vi "HTTP_Accel_Reader.vi"() -> ()   [LabVIEW 2021]
uses:
  <vilib>/myRIO/Instrument Drivers/Onboard Devices/Accelerometer/typedefs/Accelerometer Reference.ctl
  <vilib>/myRIO/Common/Instrument Driver Framework/Utilities/typedefs/myRIO Generic Hardware Reference.ctl
  <vilib>/myRIO/Common/Instrument Driver Framework/Utilities/typedefs/Hardware Version Enum.ctl
  <vilib>/myRIO/Common/Instrument Driver Framework/Utilities/typedefs/myRIO v1.0 Reference.ctl
  <vilib>/myRIO/Common/Instrument Driver Framework/Utilities/typedefs/Generic FPGA Reference.ctl
  <vilib>/myRIO/Common/Instrument Driver Framework/myRIO v1.0/Accelerometer/typedefs/Accelerometer Channels List.ctl
  <vilib>/myRIO/Common/Instrument Driver Framework/myRIO v1.0/Accelerometer/typedefs/Accelerometer Channels Enum.ctl
  <vilib>/userDefined/High Color/nirio_resource_hc.ctl
  <vilib>/myRIO/Instrument Drivers/Onboard IO/AI/typedefs/AI Reference.ctl
  <vilib>/myRIO/Common/Instrument Driver Framework/myRIO v1.0/AI/typedefs/AI Channels List.ctl
  <vilib>/myRIO/Common/Instrument Driver Framework/myRIO v1.0/AI/typedefs/AI Channels Enum.ctl
  <vilib>/myRIO/Common/Instrument Driver Framework/Utilities/typedefs/Analog Scaling Constants List.ctl
  <vilib>/myRIO/Common/Instrument Driver Framework/Utilities/typedefs/Analog Scaling Constants.ctl
  <vilib>/myRIO/Instrument Drivers/Onboard IO/DIO/typedefs/DIO Reference.ctl
  <vilib>/myRIO/Common/Instrument Driver Framework/myRIO v1.0/DIO/typedefs/DIO Channels List.ctl
  <vilib>/myRIO/Common/Instrument Driver Framework/myRIO v1.0/DIO/typedefs/DIO Channels Enum.ctl
  <vilib>/myRIO/Common/Instrument Driver Framework/Utilities/vis/Is FPGA Ref Available.vi
  <vilib>/myRIO/Common/Instrument Driver Framework/myRIO v1.0/AI/vis/myRIO v1.1 Open AI.vi
  <vilib>/myRIO/Instrument Drivers/Onboard IO/AI/vis/Read.vi
  <vilib>/myRIO/Common/Instrument Driver Framework/myRIO v1.0/Accelerometer/vis/myRIO v1.1 Open Accelerometer.vi
  <vilib>/myRIO/Instrument Drivers/Onboard Devices/Accelerometer/vis/Read.vi
  <vilib>/myRIO/Common/Instrument Driver Framework/myRIO v1.0/DIO/vis/myRIO v1.1 Open DIO.vi
  <vilib>/myRIO/Instrument Drivers/Onboard IO/DIO/vis/Write.vi
  <vilib>/myRIO/Common/Instrument Driver Framework/Utilities/vis/Validate Channels.vi
  <vilib>/myRIO/Common/Instrument Driver Framework/myRIO v1.0/AI/vis/myRIO v1.0 Reserve AI.vi
  <vilib>/myRIO/Common/Instrument Driver Framework/myRIO v1.0/Accelerometer/vis/myRIO v1.0 Reserve Accelerometer.vi
  <vilib>/myRIO/Common/Instrument Driver Framework/myRIO v1.0/DIO/vis/myRIO v1.0 Reserve DIO.vi
  <vilib>/myRIO/Common/Instrument Driver Framework/myRIO v1.0/AI/vis/myRIO v1.0 Build MUX Configuration AI.vi
  <vilib>/myRIO/Common/Instrument Driver Framework/myRIO v1.0/Resource Manager/vis/myRIO v1.0 Reserve Channel List.vi
  <vilib>/myRIO/Common/Instrument Driver Framework/myRIO v1.0/Accelerometer/vis/myRIO v1.0 Build MUX Configuration Accelerometer.vi
  <vilib>/myRIO/Common/Instrument Driver Framework/myRIO v1.0/DIO/vis/myRIO v1.0 Build MUX Configuration DIO.vi
  <vilib>/myRIO/Common/Instrument Driver Framework/myRIO v1.0/Resource Manager/vis/myRIO v1.0 Reserve Channel.vi
  <vilib>/myRIO/Common/Instrument Driver Framework/myRIO v1.0/Resource Manager/vis/myRIO v1.0 Unreserve Channel.vi
  <vilib>/myRIO/Common/Instrument Driver Framework/myRIO v1.0/Resource Manager/vis/myRIO v1.0 Create Configuration List.vi
  <vilib>/myRIO/Common/Instrument Driver Framework/myRIO v1.0/Resource Manager/vis/myRIO v1.0 Build Mutex Name.vi
  <vilib>/Utility/VariantDataType/GetNumericInfo.vi
  <vilib>/Utility/error.llb/Error Cluster From Error Code.vi
  <vilib>/myRIO/Common/Instrument Driver Framework/myRIO v1.0/myRIO v1.1 Open.vi
  <vilib>/myRIO/Common/Instrument Driver Framework/myRIO v1.0/Accelerometer/vis/myRIO v1.0 Get Scaling Constant Accelerometer.vi
  <vilib>/myRIO/Common/Instrument Driver Framework/Utilities/vis/IO Manager.vi
  <vilib>/myRIO/Common/Instrument Driver Framework/Utilities/vis/Configuration Manager.vi
  <vilib>/myRIO/Common/Instrument Driver Framework/myRIO v1.0/myRIO v1.0 Close.vi
  <vilib>/myRIO/Common/Instrument Driver Framework/myRIO v1.0/Accelerometer/vis/myRIO v1.0 Read Accelerometer.vi
  <vilib>/myRIO/Common/Instrument Driver Framework/myRIO v1.0/AI/vis/myRIO v1.0 Get Scaling Constants AI.vi
  <vilib>/myRIO/Common/Instrument Driver Framework/myRIO v1.0/AI/vis/myRIO v1.0 Read AI.vi
  <vilib>/myRIO/Common/Instrument Driver Framework/myRIO v1.0/Resource Manager/vis/myRIO v1.0 Configure IO.vi
  <vilib>/myRIO/Common/Instrument Driver Framework/myRIO v1.0/DIO/vis/myRIO v1.0 Write DIO.vi
  <vilib>/httpClient/POSTBuffer.vi
  <vilib>/myRIO/Express VI/Onboard Devices/Accelerometer/Accelerometer Express VI.xnode
  <vilib>/myRIO/Instrument Drivers/Onboard Devices/Accelerometer/vis/myRIO Accelerometer Open.xnode
  <vilib>/myRIO/Express VI/Onboard IO/AI/AI Express VI.xnode
  <vilib>/myRIO/Instrument Drivers/Onboard IO/AI/vis/myRIO AI Open.xnode
  <vilib>/myRIO/Express VI/Onboard IO/DO/DO Express VI.xnode
  <vilib>/myRIO/Instrument Drivers/Onboard IO/DIO/vis/myRIO DIO Open.xnode
  <vilib>/myRIO/Instrument Drivers/Onboard Devices/Accelerometer/Accelerometer.lvlib
  <vilib>/myRIO/Instrument Drivers/Onboard IO/DIO/DIO.lvlib
  <vilib>/httpClient/LabVIEWHTTPClient.lvlib
  <vilib>/myRIO/Instrument Drivers/Onboard IO/AI/AI.lvlib
panel:
  out "element":string
  out "Address2":string
  out "Address1":string
  in  "stop 2":bool
  out "txt":string
  out "txt 2":string
  out "error out 3":errorcluster
  out "error out 2":errorcluster
  out "A/AI3 (Pin 9)":dbl
  out "A/AI0 (Pin 3)":dbl
  out "output variable":dbl
  out "date string":string
  out "error out":errorcluster
  in  "stop":bool
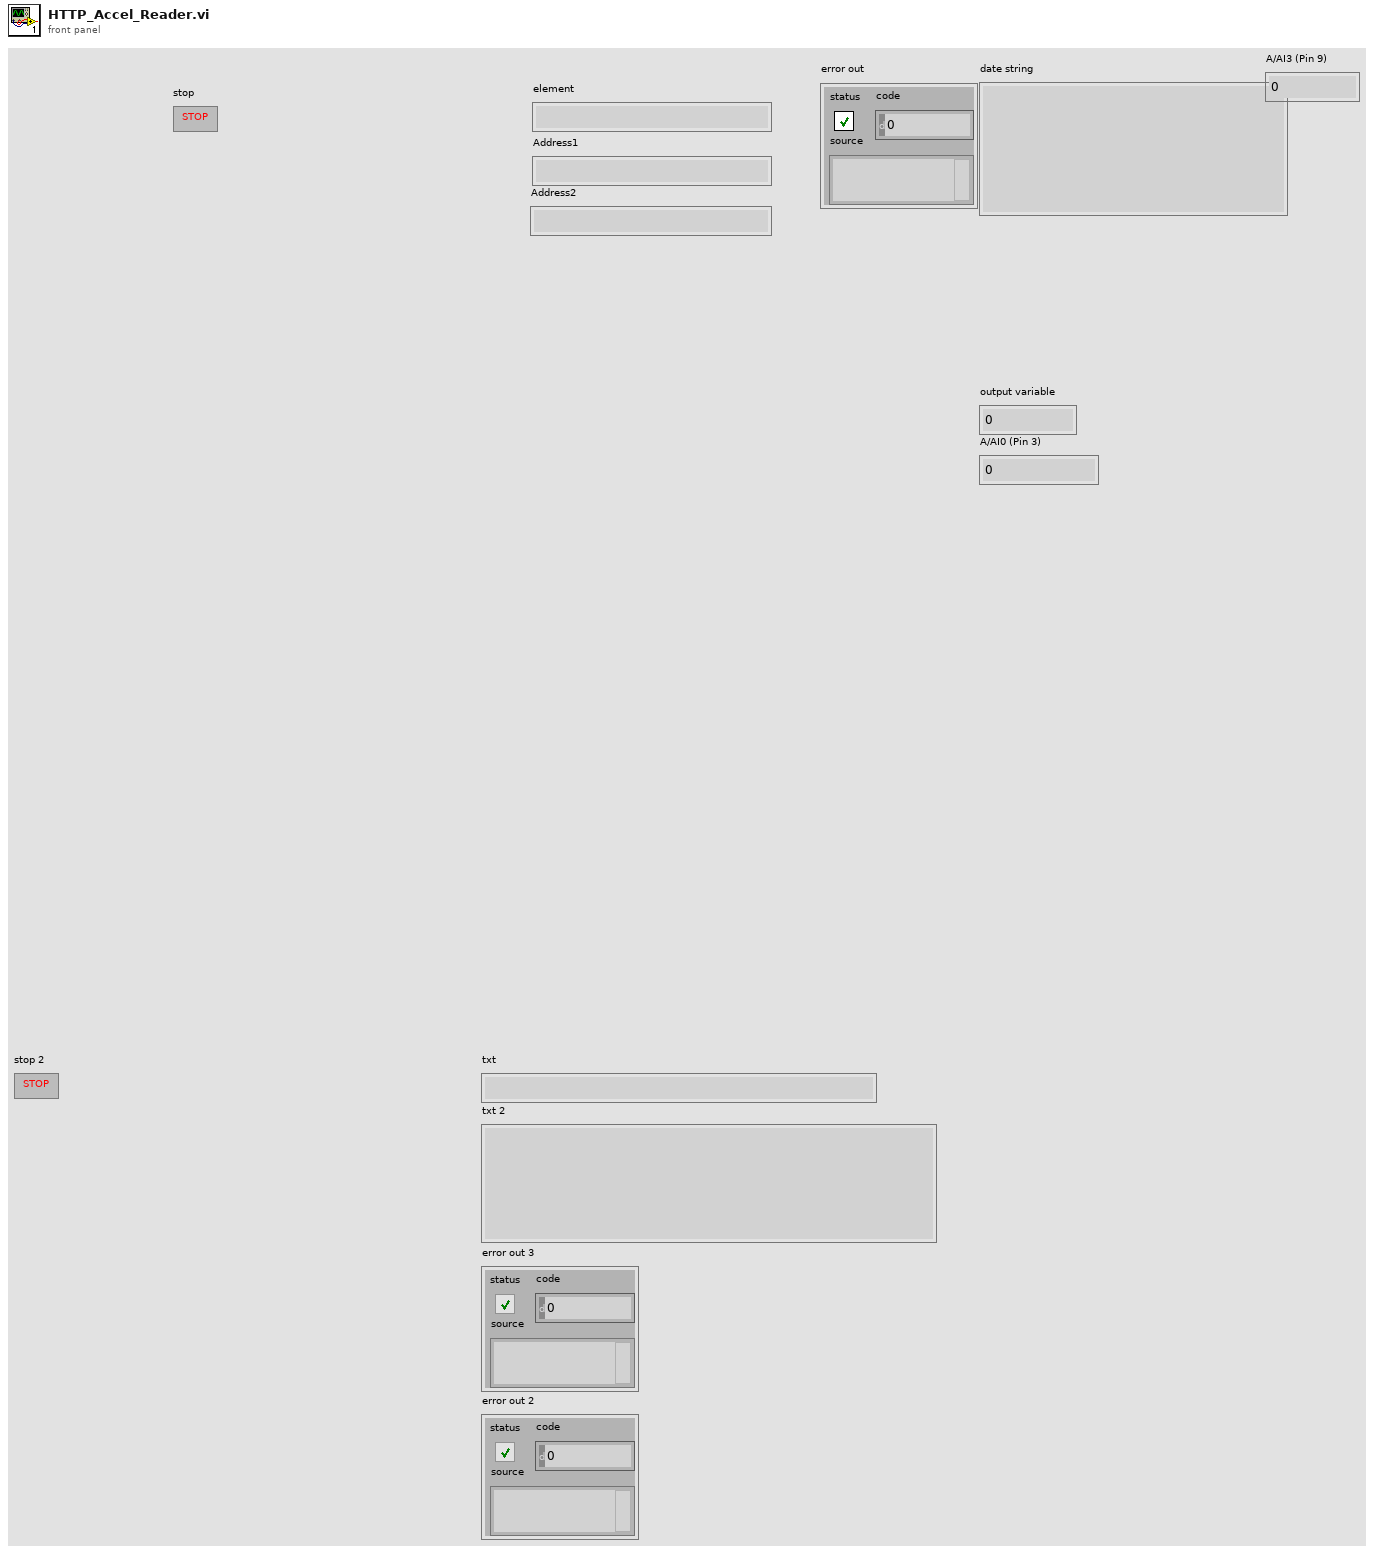
[diagram p1: front panel]
types:
  T1 = typedef "LabVIEWHTTPClient.lvlib/ClientHandle.ctl" = refnum<k1>
  T2 = typedef "DIO.lvlib/DIO Reference.ctl" = cluster{"myRIO Reference":T3, "DIO Channels List":T7}
  T3 = typedef "myRIO Generic Hardware Reference.ctl" = cluster{"myRIO Model":T4, "myRIO Hardware Reference":T5}
  T4 = typedef "Hardware Version Enum.ctl" = enum16{"Unknown", "myRIO-1900", "myRIO-1950", "roboRIO", "NI ELVIS RIO CM", "ELVIS III"}
  T5 = typedef "myRIO v1.0 Reference.ctl" = cluster{"Generic FPGA Reference":T6, "Allow multiple opens":bool}
  T6 = typedef "Generic FPGA Reference.ctl" = refnum<k20>
  T7 = typedef "DIO Channels List.ctl" = T8[]
  T8 = typedef "DIO Channels Enum.ctl" = enum16{"Not Connected", "C/DIO0", "C/DIO1", "C/DIO2", "C/DIO3", "C/DIO4", "C/DIO5", "C/DIO6", "C/DIO7", "A/DIO0", "A/DIO1", "A/DIO2", "A/DIO3", "A/DIO4", "A/DIO5", "A/DIO6", "A/DIO7", "A/DIO8", "A/DIO9", "A/DIO10", "A/DIO11", "A/DIO12", "A/DIO13", "A/DIO14", "A/DIO15", "A/DIO16", "A/DIO17", "A/DIO18", "A/DIO19", "B/DIO0", "B/DIO1", "B/DIO2", "B/DIO3", "B/DIO4", "B/DIO5", "B/DIO6", "B/DIO7", "B/DIO8", "B/DIO9", "B/DIO10", "B/DIO11", "B/DIO12", "B/DIO13", "B/DIO14", "B/DIO15", "B/DIO16", "B/DIO17", "B/DIO18", "B/DIO19", "LED0", "LED1", "LED2", "LED3", "Button0", "DIO/DIO0", "DIO/DIO1", "DIO/DIO2", "DIO/DIO3", "DIO/DIO4", "DIO/DIO5", "DIO/DIO6", "DIO/DIO7", "DIO/DIO8", "DIO/DIO9", "SPI/CS0", "SPI/CS1", "SPI/CS2", "SPI/CS3", "LED RADIO (Green)", "LED RADIO (Red)", "LED COMM (Green)", "LED COMM (Red)", "LED MODE (Green)", "LED MODE (Red)"}
  T9 = typedef "nirio_resource_hc.ctl" = tag
  T10 = typedef "AI.lvlib/AI Reference.ctl" = cluster{"myRIO Reference":T3, "AI Channels List":T11, "AI Scaling Constants List":T13}
  T11 = typedef "AI Channels List.ctl" = T12[]
  T12 = typedef "AI Channels Enum.ctl" = enum16{"Not Connected", "AudioIn/Left", "AudioIn/Right", "C/AI0", "C/AI1", "A/AI0", "A/AI1", "A/AI2", "A/AI3", "A/AI4", "A/AI5", "A/AI6", "A/AI7", "B/AI0", "B/AI1", "B/AI2", "B/AI3", "B/AI4", "B/AI5", "B/AI6", "B/AI7", "AI/AI0", "AI/AI1", "AI/AI2", "AI/AI3", "A/AI0 (DIFF)", "A/AI1 (DIFF)", "A/AI2 (DIFF)", "A/AI3 (DIFF)", "B/AI0 (DIFF)", "B/AI1 (DIFF)", "B/AI2 (DIFF)", "B/AI3 (DIFF)"}
  T13 = typedef "Analog Scaling Constants List.ctl" = T14[]
  T14 = typedef "Analog Scaling Constants.ctl" = cluster{"LSB Weight (Volts)":dbl, "Offset (Volts)":dbl, "Signed?":bool}
  T15 = typedef "Accelerometer.lvlib/Accelerometer Reference.ctl" = cluster{"myRIO Reference":T3, "Accelerometer Channels List":T16, "LSB Weight":dbl}
  T16 = typedef "Accelerometer Channels List.ctl" = T17[]
  T17 = typedef "Accelerometer Channels Enum.ctl" = enum16{"Not Connected", "X-Axis", "Y-Axis", "Z-Axis"}
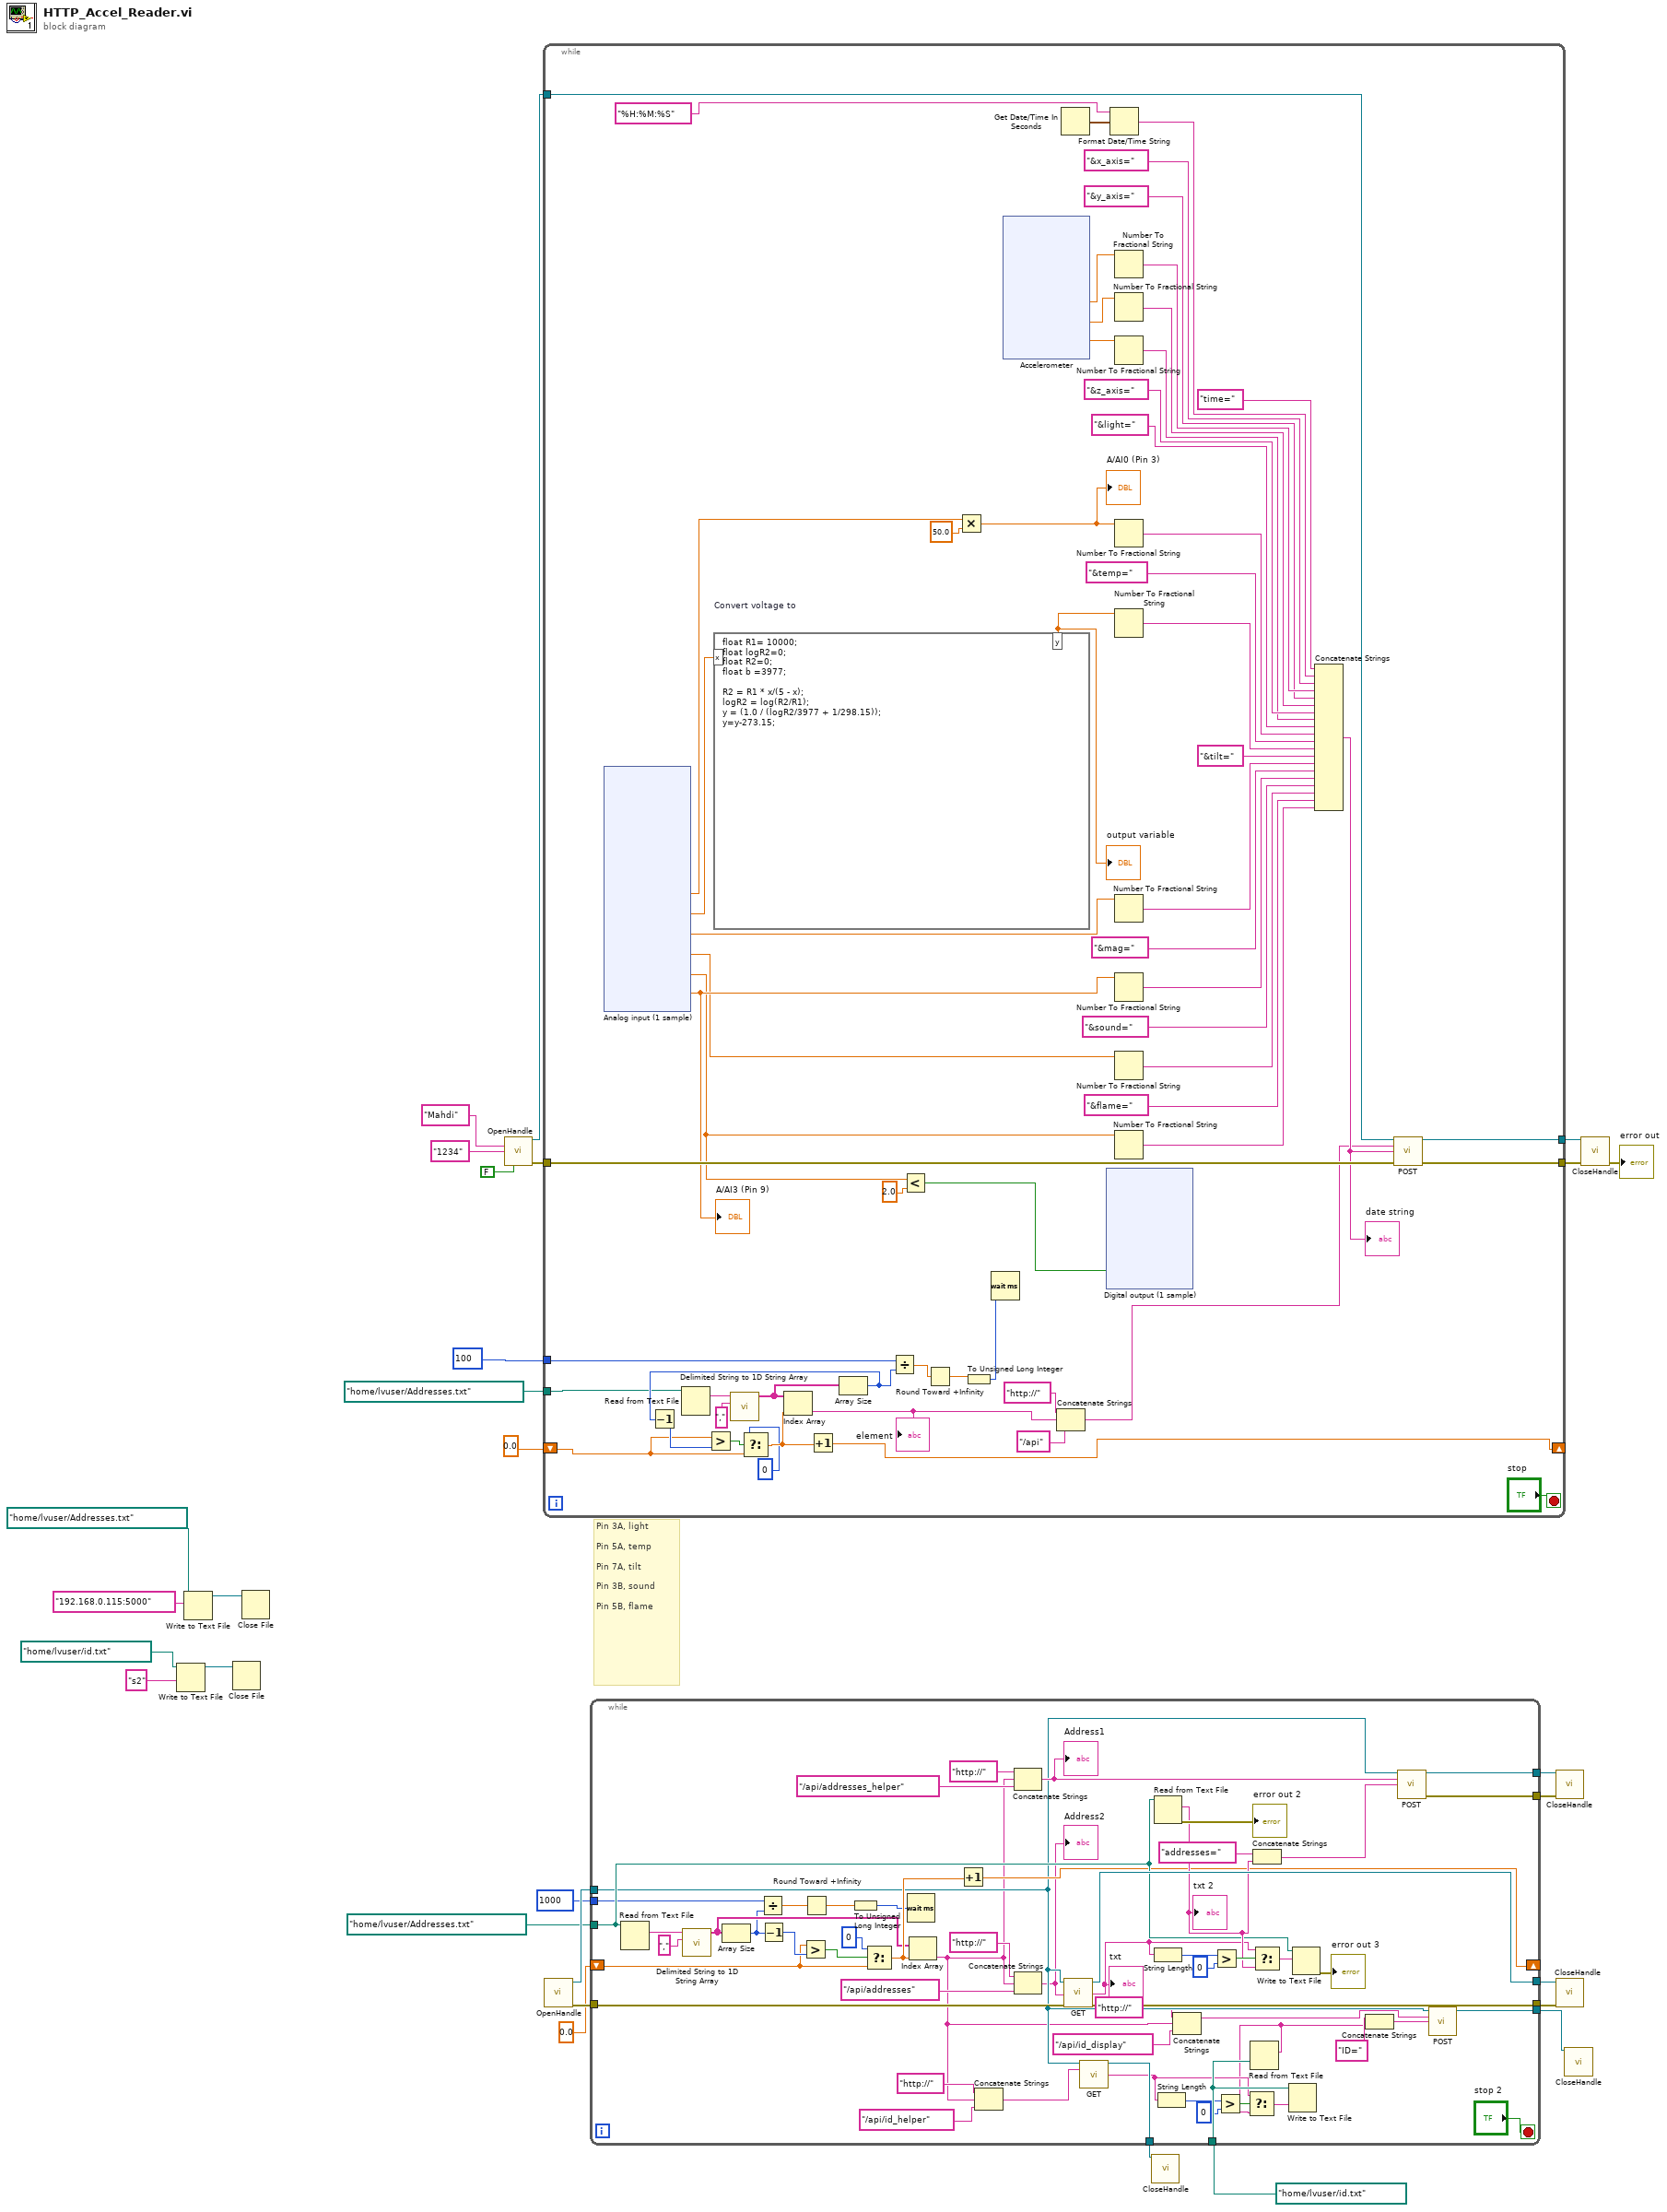
[diagram p0: block diagram]
diagram:
  # "Pin 3A, light\n\nPin 5A, temp\n\nPin 7A, tilt\n\nPin 3B, sound\n\nPin 5B, flame"
  n1 = Write to Text File(file (use dialog)=path "/home/lvuser/id.txt" ("file path (use dialog)"), text="s2") -> (refnum out=w3:refnum<file>)  [unwired: 2 in, 2 out]
  n2 = Write to Text File(file (use dialog)=path "/home/lvuser/Addresses.txt" ("file path (use dialog)"), text="192.168.0.115:5000") -> (refnum out=w4:refnum<file>)  [unwired: 2 in, 2 out]
  n3 = Close File(refnum=w3) -> ()  [unwired: 1 in, 2 out]
  n4 = Close File(refnum=w4) -> ()  [unwired: 1 in, 2 out]
  n5 = call <vilib>:"OpenHandle.vi"("username"="Mahdi", "password"="1234", "verify server(true)"=FALSE) -> ("client handle out"=w27:T1, "error out"=w26:errorcluster)  [unwired: 11 in]
  n6 = while {
    tunnel: w27 -> [w81]
    tunnel: w26 -> [w78]
    tunnel: [w79] -> w23
    tunnel: [w80] -> w24
    tunnel: u32 100 ("millisecond timer value") -> [w34]
    tunnel: path "/home/lvuser/Addresses.txt" ("file path (use dialog)") -> [w33]
    shift-right: [w31] -> _
    shift-left: 0.0 -> [w32]
    stop <- "stop" stop-if-true
    n7 = xnode "Analog input (1 sample)"() -> ("A/AI0 (Pin 3)"=w63:dbl, "A/AI1 (Pin 5)"=w64:dbl, "A/AI2 (Pin 7)"=w60:dbl, "B/AI0 (Pin 3)"=w55:dbl, "B/AI1 (Pin 5)"=w51:dbl, "A/AI3 (Pin 9)"=w57:dbl)  [unwired: 1 in, 1 out]
    "A/AI3 (Pin 9)" <- w57
    n8 = Read from Text File(file (use dialog)=w33) -> (text=w41:string)  [unwired: 3 in, 3 out]
    n9 = formula code="float R1= 10000; \nfloat logR2=0; \nfloat R2=0;\nfloat b =3977;\n\nR2 = R1 * x/(5 - x); \nlogR2 = log(R2/R1);\ny = (1.0 / (logR2/3977 + 1/298.15)); \ny=y-273.15;" "Convert voltage to"("x"=w64) -> ("y"=w69:dbl)
    "output variable" <- w69
    n10 = call <vilib>:"Delimited String to 1D String Array.vi"("delimiter"=",", "delimited string"=w41) -> ("string array"=w43:string[])  [unwired: 9 in]
    n11 = Array Size(array=w43) -> (size(s)=w35:i32)
    n12 = Decrement(x=w35) -> (x-1=w47:i32)
    n13 = Greater?(x=w32, y=w47) -> (0:w46:bool)
    n14 = Select(t=u32 0, s=w46, f=w32) -> (s? t:f=w48:dbl)
    n15 = Index Array(array=w43, index=w48) -> (element=w42:string)
    "element" <- w42
    n16 = Increment(x=w48) -> (x+1=w31:dbl)
    n17 = Divide(x=w34, y=w35) -> (x/y=w45:dbl)
    n18 = Less?(x=w51, y=2.0) -> (x < y?=w49:bool)
    n19 = Round Toward +Infinity(x=w45) -> (ceil(x): smallest int >= x=w44:dbl)
    n20 = Multiply(x=w63, y=50.0) -> (x*y=w70:dbl)
    "A/AI0 (Pin 3)" <- w70
    n21 = To Unsigned Long Integer(number=w44) -> (unsigned 32bit integer=w36:u32)
    n22 = Wait (ms)(milliseconds to wait=w36) -> ()  [unwired: 1 out]
    n23 = xnode "Accelerometer"() -> ("X-Axis"=w85:dbl, "Y-Axis"=w86:dbl, "Z-Axis"=w87:dbl)  [unwired: 1 in, 1 out]
    n24 = Concatenate Strings("http://" ("string"), w42, "/api" ("string")) -> (w30:string)
    n25 = Get Date/Time In Seconds() -> (seconds since 1Jan1904=w75:timestamp)
    n26 = xnode "Digital output (1 sample)"("B/DIO0 (Pin 11)"=w49) -> ()  [unwired: 1 in, 1 out]
    n27 = Format Date/Time String(time format string (%c)="%H:%M:%S", seconds (now)=w75) -> (date/time string=w74:string)  [unwired: 1 in]
    n28 = Number To Fractional String(number=w85) -> (F-format string=w88:string)  [unwired: 3 in]
    n29 = Number To Fractional String(number=w86) -> (F-format string=w89:string)  [unwired: 3 in]
    n30 = Number To Fractional String(number=w87) -> (F-format string=w72:string)  [unwired: 3 in]
    n31 = Number To Fractional String(number=w70) -> (F-format string=w67:string)  [unwired: 3 in]
    n32 = Number To Fractional String(number=w69) -> (F-format string=w66:string)  [unwired: 3 in]
    n33 = Number To Fractional String(number=w60) -> (F-format string=w61:string)  [unwired: 3 in]
    n34 = Number To Fractional String(number=w57) -> (F-format string=w58:string)  [unwired: 3 in]
    n35 = Number To Fractional String(number=w55) -> (F-format string=w54:string)  [unwired: 3 in]
    n36 = Number To Fractional String(number=w51) -> (F-format string=w53:string)  [unwired: 3 in]
    n37 = Concatenate Strings("time=" ("string"), w74, "&x_axis=", w88, "&y_axis=", w89, "&z_axis=", w72, "&light=", w67, "&temp=", w66, "&tilt=", w61, "&mag=", w58, "&sound=", w54, "&flame=", w53) -> (w76:string)
    "date string" <- w76
    n38 = call-poly <vilib>:"POST.vi"("client handle"=w81, "url"=w30, "buffer"=w76, "error in (no error)"=w78) -> ("client handle out"=w80:T1, "error out"=w79:errorcluster)  [unwired: 8 in, 2 out]
  }
  n39 = call <vilib>:"OpenHandle.vi"() -> ("client handle out"=w21:T1, "error out"=w20:errorcluster)  [unwired: 14 in]
  n40 = while {
    tunnel: path "/home/lvuser/Addresses.txt" ("file path (use dialog)") -> [w235]
    tunnel: w21 -> [w221]
    tunnel: w20 -> [w261]
    tunnel: [w260] -> w19
    tunnel: [w259] -> w18
    tunnel: [w258] -> w17
    tunnel: [w257] -> w16
    tunnel: u32 1000 ("millisecond timer value") -> [w234]
    shift-right: [w230] -> _
    shift-left: 0.0 -> [w231]
    tunnel: path "/home/lvuser/id.txt" ("file path (use dialog)") -> [w228]
    tunnel: [w222] -> w8
    tunnel: [w220] -> w7
    stop <- "stop 2" stop-if-true
    n41 = Read from Text File(file (use dialog)=w235) -> (text=w242:string)  [unwired: 3 in, 3 out]
    n42 = call <vilib>:"Delimited String to 1D String Array.vi"("delimiter"=",", "delimited string"=w242) -> ("string array"=w243:string[])  [unwired: 9 in]
    n43 = Array Size(array=w243) -> (size(s)=w229:i32)
    n44 = Divide(x=w234, y=w229) -> (x/y=w245:dbl)
    n45 = Decrement(x=w229) -> (x-1=w247:i32)
    n46 = Greater?(x=w231, y=w247) -> (0:w246:bool)
    n47 = Round Toward +Infinity(x=w245) -> (ceil(x): smallest int >= x=w244:dbl)
    n48 = To Unsigned Long Integer(number=w244) -> (unsigned 32bit integer=w233:u32)
    n49 = Select(t=u32 0, s=w246, f=w231) -> (s? t:f=w248:dbl)
    n50 = Wait (ms)(milliseconds to wait=w233) -> ()  [unwired: 1 out]
    n51 = Index Array(array=w243, index=w248) -> (element=w209:string)
    n52 = Increment(x=w248) -> (x+1=w230:dbl)
    n53 = Concatenate Strings("http://" ("string"), w209, "/api/id_helper" ("string")) -> (w213:string)
    n54 = Concatenate Strings("http://" ("string"), w209, "/api/addresses_helper" ("string")) -> (w232:string)
    "Address1" <- w232
    n55 = Concatenate Strings("http://" ("string"), w209, "/api/addresses" ("string")) -> (w214:string)
    "Address2" <- w214
    n56 = call <vilib>:"GET.vi"("client handle"=w221, "url"=w214, "error in (no error)"=w261) -> ("client handle out"=w259:T1, "body"=w226:string, "error out"=w260:errorcluster)  [unwired: 9 in, 1 out]
    "txt" <- w226
    n57 = call <vilib>:"GET.vi"("client handle"=w221, "url"=w213) -> ("client handle out"=w220:T1, "body"=w215:string)  [unwired: 10 in, 2 out]
    n58 = Read from Text File(file (use dialog)=w235) -> (text=w249:string, error out=→"error out 2":errorcluster)  [unwired: 3 in, 2 out]
    "txt 2" <- w249
    n59 = String Length(string=w226) -> (length=w252:i32)
    n60 = String Length(string=w215) -> (length=w219:i32)
    n61 = Concatenate Strings("http://" ("string"), w209, "/api/id_display" ("string")) -> (w210:string)
    n62 = Greater?(x=w252, y=0) -> (0:w251:bool)
    n63 = Greater?(x=w219, y=0) -> (0:w218:bool)
    n64 = Read from Text File(file (use dialog)=w228) -> (text=w207:string)  [unwired: 3 in, 3 out]
    n65 = Select(t=w215, s=w218, f=w207) -> (s? t:f=w216:string)
    n66 = Concatenate Strings("addresses=" ("string"), w249) -> (w255:string)
    n67 = Select(t=w226, s=w251, f=w249) -> (s? t:f=w227:string)
    n68 = Write to Text File(file (use dialog)=w228, text=w216) -> ()  [unwired: 2 in, 3 out]
    n69 = Write to Text File(file (use dialog)=w235, text=w227) -> (error out=→"error out 3":errorcluster)  [unwired: 2 in, 2 out]
    n70 = Concatenate Strings("ID=" ("string"), w207) -> (w223:string)
    n71 = call-poly <vilib>:"POST.vi"("client handle"=w221, "url"=w232, "buffer"=w255) -> ("client handle out"=w257:T1, "error out"=w258:errorcluster)  [unwired: 9 in, 2 out]
    n72 = call-poly <vilib>:"POST.vi"("client handle"=w221, "url"=w210, "buffer"=w223) -> ("client handle out"=w222:T1)  [unwired: 9 in, 3 out]
  }
  n73 = call <vilib>:"CloseHandle.vi"("client handle"=w7) -> ()  [unwired: 14 in, 1 out]
  n74 = call <vilib>:"CloseHandle.vi"("client handle"=w16, "error in (no error)"=w17) -> ()  [unwired: 13 in, 1 out]
  n75 = call <vilib>:"CloseHandle.vi"("client handle"=w18, "error in (no error)"=w19) -> ()  [unwired: 13 in, 1 out]
  n76 = call <vilib>:"CloseHandle.vi"("client handle"=w8) -> ()  [unwired: 14 in, 1 out]
  n77 = call <vilib>:"CloseHandle.vi"("client handle"=w24, "error in (no error)"=w23) -> ("error out"=→"error out":errorcluster)  [unwired: 13 in]
